vi "SaveImage.vi"(8 "Error In":errorcluster, 10 "Image In":T1[](array[typedef]), 11 "Snapshot images folder path":path) -> (0 "Error Out":errorcluster)   [LabVIEW 2013]
uses:
  <vilib>/vision/Image Controls.llb/IMAQ Image.ctl
  <vilib>/vision/NI_Vision_Development_Module.lvlib
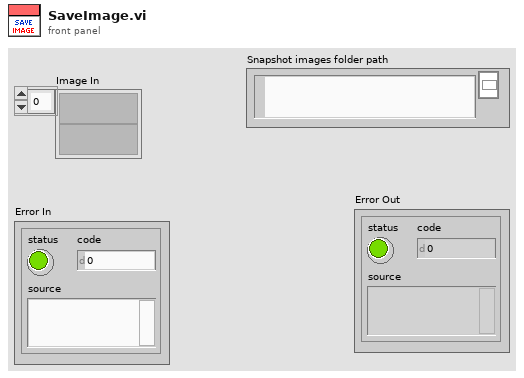
[diagram p1: front panel]
types:
  T1 = typedef "IMAQ Image.ctl" = refnum<image>
  T2 = typedef "Image Type" = u32
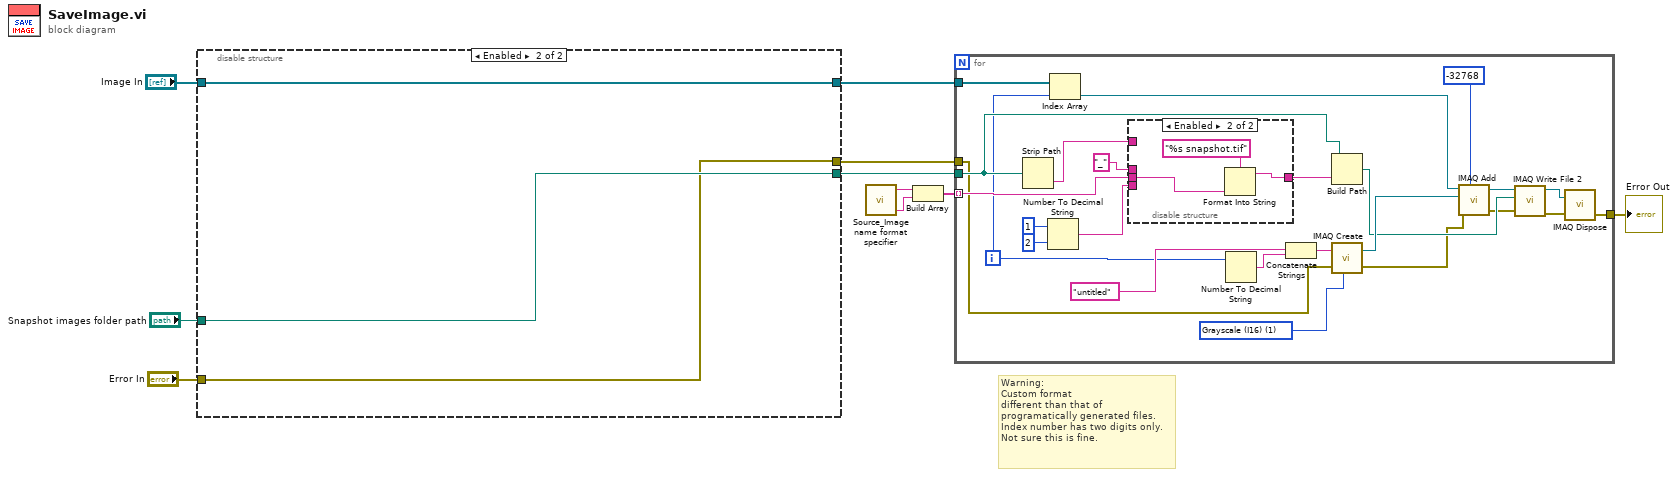
[diagram p0: block diagram]
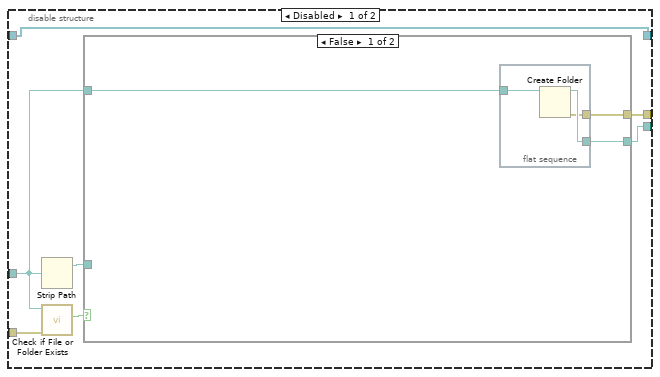
[diagram p2: hidden frame]
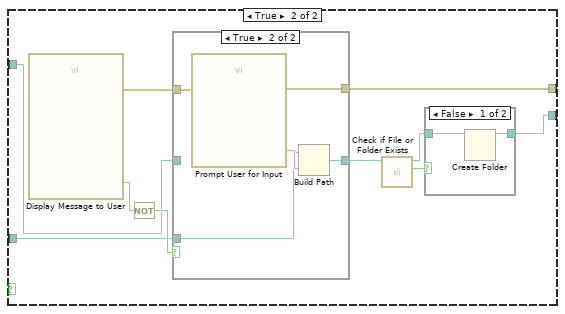
[diagram p3: hidden frame]
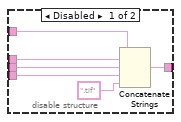
[diagram p6: hidden frame]
diagram:
  # "Warning:\nCustom format\ndifferent than that of programatically generated files.\nIndex number has two digits only. Not sure this is fine."
  n1 = disable-structure shown="Enabled" {
    disable-tunnel: "Snapshot images folder path" -> [w15 w46]
    disable-tunnel: [w14 w46] -> w2
    disable-tunnel: [w13 w45] -> w1
    disable-tunnel: "Error In" -> [w12 w45]
    disable-tunnel: "Image In" -> [w11 w44]
    disable-tunnel: [w11 w44] -> w3
    frame Disabled {
      n2 = Strip Path(path=w15) -> (stripped path=w16:path)  [unwired: 1 out]
      n3 = call <vilib>:"Check if File or Folder Exists.vi"("error in (no error)"=w12, "path"=w15) -> ("file or folder exists?"=w17:bool)  [unwired: 7 in, 2 out]
      n4 = case shown="False" w17 {
        tunnel: [w20 w24] -> w14
        tunnel: w16 -> [_ w28]
        tunnel: [w19 w30] -> w13
        tunnel: w15 -> [w18 w29]
        frame False {
          n5 = flat-sequence {
            tunnel: [w22] -> w20
            tunnel: w18 -> [w23]
            tunnel: [w21] -> w19
            frame #0 {
              n6 = Create Folder(path (use dialog)=w23) -> (created path=w22:path, error out=w21:errorcluster)  [unwired: 2 in, 1 out]
            }
          }
        }
        frame True {
          n7 = call "Display Message to User"() -> ("error out"=w33:errorcluster, "Overwrite"=w32:bool)  [unwired: 10 in]
          n8 = Not(x=w32) -> (.not. x?=w31:bool)
          n9 = case shown="True" w31 {
            tunnel: [w37 w42] -> w27
            tunnel: w29 -> [w37 _]
            tunnel: w33 -> [w38 w41]
            tunnel: [w38 w40] -> w30
            tunnel: w28 -> [_ w39]
            frame False {
            }
            frame True {
              n10 = call "Prompt User for Input"("error in (no error)"=w41) -> ("Folder Name"=w43:string, "error out"=w40:errorcluster)  [unwired: 16 in, 1 out]
              n11 = Build Path(base path=w39, name or relative path=w43) -> (appended path=w42:path)
            }
          }
          n12 = call <vilib>:"Check if File or Folder Exists.vi"("path"=w27) -> ("file or folder exists?"=w25:bool, "dup path"=w26:path)  [unwired: 8 in, 1 out]
          n13 = case shown="False" w25 {
            tunnel: w26 -> [w35 w36]
            tunnel: [w34 w36] -> w24
            frame False {
              n14 = Create Folder(path (use dialog)=w35) -> (created path=w34:path)  [unwired: 2 in, 2 out]
            }
            frame True {
            }
          }
        }
      }
    }
    frame Enabled {
    }
  }
  n15 = call "Source_Image name format specifier.vi"() -> ("Red channel name"=w6:string, "Green channel name"=w5:string)  [unwired: 5 in, 1 out]
  n16 = Build Array(w6, w5) -> (w7:string[])
  n17 = for {
    tunnel: w2 -> [w56]
    tunnel: w1 -> [w53]
    tunnel: w3 -> [w50]
    tunnel: w7 -> [w69] mode=indexing
    tunnel: [w58] -> w8
    i -> [w47]
    w71 = T2 1 items=["Grayscale (U8)", "Grayscale (I16)", "Grayscale (SGL)", "Complex (CSG)", "RGB (U32)", "HSL (U32)", "RGB (U64)"] ("Image Type")
    n18 = Strip Path(path=w56) -> (name=w55:string)  [unwired: 1 out]
    n19 = Number To Decimal String(number=1 ("x"), width (-)=i16 2) -> (decimal integer string=w65:string)
    n20 = Index Array(array=w50, index=w47) -> (element=w49:T1)
    n21 = disable-structure shown="Enabled" {
      disable-tunnel: w69 -> [w77 w79]
      disable-tunnel: [w75 w78] -> w67
      disable-tunnel: w65 -> [w74 _]
      disable-tunnel: w55 -> [w73 _]
      disable-tunnel: "_" ("string") -> [w72 _]
      frame Disabled {
        n22 = Concatenate Strings(w73, w72, w77, w74, ".tif" ("string")) -> (w75:string)
      }
      frame Enabled {
        n23 = Format Into String(format string="%s snapshot.tif", w79) -> (resulting string=w78:string)  [unwired: 2 in, 1 out]
      }
    }
    n24 = Number To Decimal String(number=w47) -> (decimal integer string=w62:string)  [unwired: 1 in]
    n25 = Concatenate Strings("untitled" ("Image Name"), w62) -> (w61:string)
    n26 = Build Path(base path=w56, name or relative path=w67) -> (appended path=w68:path)
    n27 = call "IMAQ Create"("Image Name"=w61, "Image Type"=w71, "error in (no error)"=w53) -> ("New Image"=w70:T1, "error out"=w52:errorcluster)  [unwired: 2 in]
    n28 = call "IMAQ Add"("Image Src A"=w49, "Constant"=i16 -32768, "Image Dst"=w70, "error in (no error)"=w52) -> ("Image Dst Out"=w64:T1, "error out"=w51:errorcluster)  [unwired: 3 in]
    n29 = call-poly "IMAQ Write File 2"("error in (no error)"=w51, "File Path"=w68, "Image"=w64) -> ("error out"=w59:errorcluster, "Image Out (duplicate)"=w60:T1)  [unwired: 7 in]
    n30 = call "IMAQ Dispose"("Image"=w60, "error in (no error)"=w59) -> ("error out"=w58:errorcluster)  [unwired: 4 in]
  }
  "Error Out" <- w8
